vi "clFile_readFromFile.vi"(10 "file (use dialog)":path) -> (2 "clFileReader.lvclass":refnum<class "clFileReader.lvclass">, 3 "clFile.lvclass":refnum<class "clFile.lvclass">)   [LabVIEW 2011, in "vi_lib.lvlib" / "clFile.lvclass"]
uses:
  clFile.lvclass
  clFileReader/clFileReader.lvclass
  clFile.lvclass/clFile.ctl
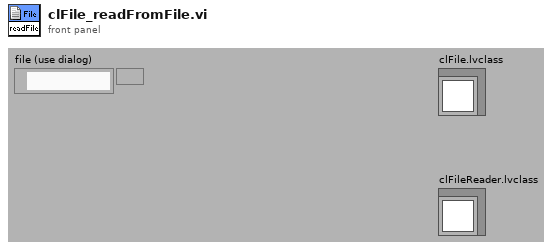
[diagram p1: front panel]
types:
  T1 = enum16{"open", "replace", "create", "open or create", "replace or create", "replace or create with confirmation"}
  T2 = enum16{"deny read/write", "deny write-only", "deny none"}
  T3 = enum16{"big-endian, network order", "native, host order", "little-endian"}
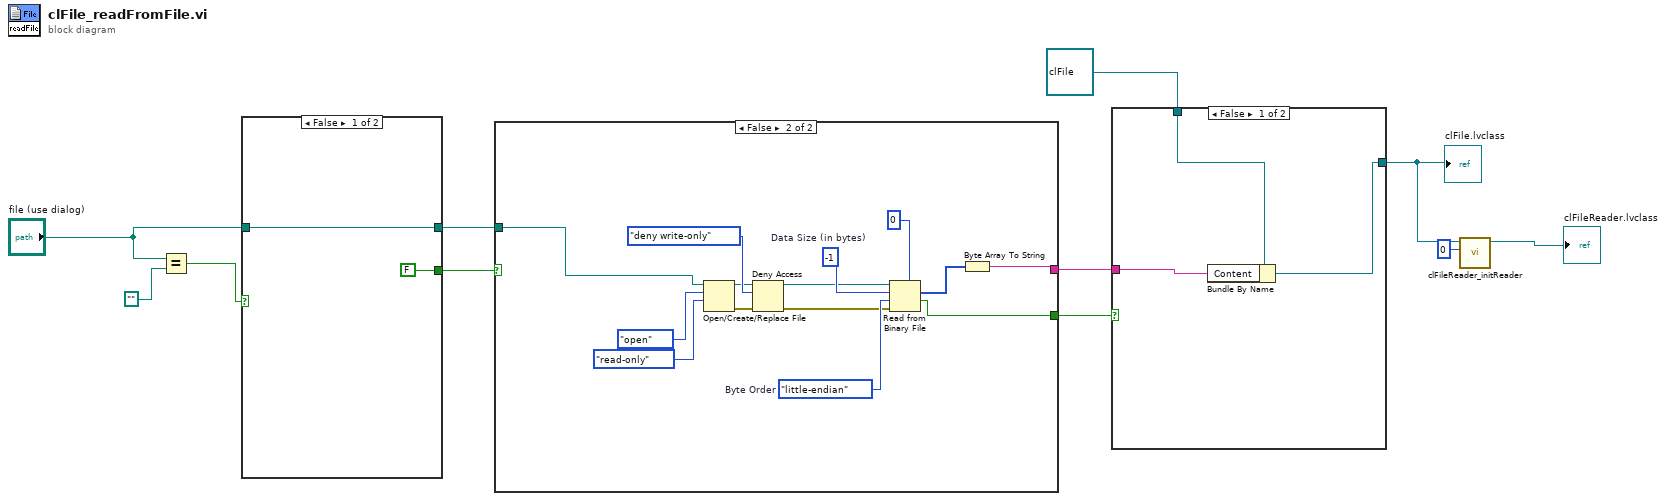
[diagram p0: block diagram]
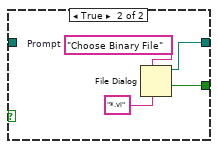
[diagram p2: hidden frame]
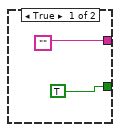
[diagram p3: hidden frame]
diagram:
  n1 = Equal?(x="file (use dialog)", y=path "") -> (x = y?=w8:bool)
  n2 = case shown="False" w8 {
    tunnel: [w13 w16] -> w6
    tunnel: "file (use dialog)" -> [w13 _]
    tunnel: [FALSE ("cancelled") w15] -> w5
    frame False {
    }
    frame True {
      w14 = "Choose Binary File"  # Prompt
      n3 = File Dialog(6:"*.vi" ("pattern (all files)"), 7:w14) -> (1:w15:bool, 3:w16:path)  [unwired: 1 in, 6 out]
    }
  }
  n4 = case shown="False" w5 {
    tunnel: [TRUE ("cancelled") w25] -> w10
    tunnel: ["" w21] -> w9
    tunnel: w6 -> [_ w20]
    frame True {
    }
    frame False {
      w27 = T3."little-endian"  # Byte Order
      w33 = i64 -1  # Data Size (in bytes)
      n5 = Open/Create/Replace File(file path (use dialog)=w20, operation (0:open)=T1."open", access (0:read/write)=enum16{"read/write", "read-only", "write-only"}."read-only") -> (refnum out=w29:refnum<file>, error out=w28:errorcluster)  [unwired: 1 in, 3 out]
      n6 = Deny Access(4:w28, 6:T2."deny write-only" ("deny mode (0:deny read/write)"), 7:w29) -> (0:w24:errorcluster, 3:w32:refnum<file>)
      n7 = Read from Binary File(5:u8 0, 8:w24, 9:w27, 10:w33, 11:w32) -> (1:w25:bool, 2:w22:u8[])  [unwired: 3 out]
      n8 = Byte Array To String(unsigned byte array=w22) -> (string=w21:string)
    }
  }
  n9 = case shown="False" w10 {
    tunnel: w9 -> [w36 _]
    tunnel: refnum<class "clFile.lvclass"> refnum ("clFile.lvclass") -> [w35 w37]
    tunnel: [w34 w37] -> w3
    frame False {
      n10 = Bundle By Name(cluster=w35, "Content"=w36) -> (w34:refnum<class "clFile.lvclass">)
    }
    frame True {
    }
  }
  "clFile.lvclass" <- w3
  n11 = call "clFileReader_initReader.vi"("HiddenOffset"=u32 0, "clFile.lvclass"=w3) -> ("clFileReader.lvclass"=→"clFileReader.lvclass":refnum<class "clFileReader.lvclass">)  [unwired: 1 in, 8 out]
